vi "Test Array to Map (Cluster of Arrays).vi"() -> ()   [LabVIEW 2020]
uses:
  9a7eb577-90c4-4537-9fff-6973843e9f2b.vi
  9a7eb577-90c4-4537-9fff-6973843e9f2b.vi/b0178052-0c48-4c9a-874f-40b592e34ac5.vi
  <vilib>/addons/_JKI Toolkits/Caraya/classes/Assert/Assert Equal Value and Type_Variant.vi
  <vilib>/addons/_JKI Toolkits/Caraya/classes/Test/Test.lvclass
  <vilib>/addons/_JKI Toolkits/Caraya/classes/Assert/Assert.lvclass
panel:
  out "error out":errorcluster
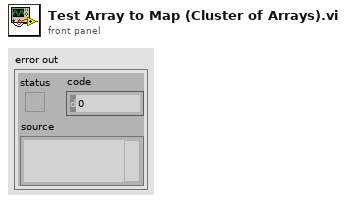
[diagram p1: front panel]
types:
  T1 = cluster{i32[], cluster{"bool":bool, "string":string}[]}
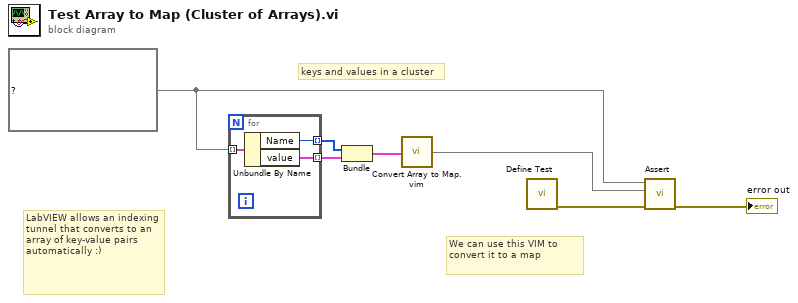
[diagram p0: block diagram]
diagram:
  w7 = map{i32, cluster{"bool":bool, "string":string}} {0={"bool"=FALSE, "string"="zero"}, 1={"bool"=TRUE, "string"="one"}} ("map out")
  # "keys and values in a cluster"
  # "We can use this VIM to convert it to a map"
  # "LabVIEW allows an indexing tunnel that converts to an array of key-value pairs automatically :)"
  n1 = for {
    tunnel: w7 -> [w10] mode=indexing
    tunnel: [w9] -> w3 mode=indexing
    tunnel: [w8] -> w2 mode=indexing
    n2 = Unbundle By Name(w10) -> ("Name"=w9:i32, "value"=w8:cluster{"bool":bool, "string":string})
  }
  n3 = Bundle(w3, w2) -> (w1:T1)  [unwired: 1 in]
  n4 = call "Convert Array to Map.vim"("array"=w1) -> ("map"=w4:map{i32, cluster{"bool":bool, "string":string}})  [unwired: 6 in]
  n5 = call <vilib>:"Define Test.vi"() -> ("error out"=w5:errorcluster)  [unwired: 11 in]
  n6 = call-poly <vilib>:"Assert.vi"("error in (no error)"=w5, "Y"=w4, "X"=w7) -> ("error out"=→"error out":errorcluster)  [unwired: 8 in]
